vi "ToDatagram.vi"(8 "error in (no error)":errorcluster, 10 "messageID":u16, 11 "PublishMqttMsg in":refnum<class "PublishMqttMsg.lvclass">) -> (0 "error out":errorcluster, 2 "Datagram":u8[](array[numeric]), 3 "PublishMqttMsg out":refnum<class "PublishMqttMsg.lvclass">)   [LabVIEW 2020, in "PublishMqttMsg.lvclass"]
uses:
  PublishMqttMsg.lvclass
  PublishMqttMsg.lvclass/PublishMqttMsg.ctl
  mqttTypedef/mqttMessageType.ctl
  mqtt.lvclass
  BaseMqttMsg.lvclass
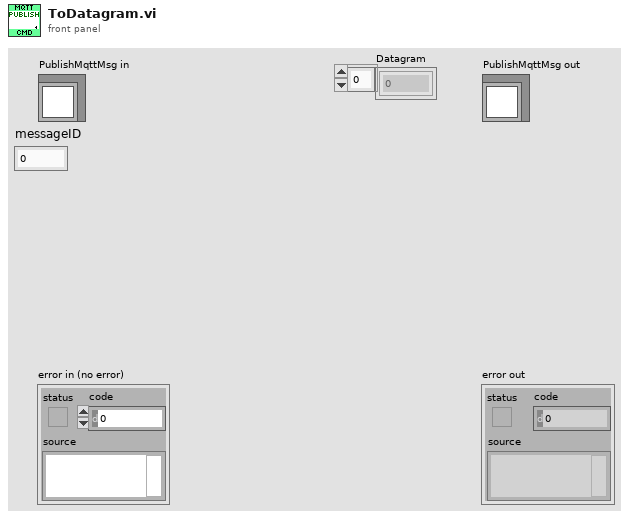
[diagram p1: front panel]
types:
  T1 = typedef "mqtt.lvclass/mqttConnectionMeta.ctl" = cluster{"qos":T2, "duplicate":bool, "retain":bool}
  T2 = typedef "mqtt.lvclass/mqttQOSlevel.ctl" = enum8{"At most once", "At least once", "Exactly once", "Reserved"}
  T3 = typedef "mqtt.lvclass/mqttMessageType.ctl" = enum32{"Reserved", "CONNECT", "CONNACK", "PUBLISH", "PUBACK", "PUBREC", "PUBREL", "PUBCOMP", "SUBSCRIBE", "SUBACK", "UNSUBSCRIBE", "UNSUBACK", "PINGREQ", "PINGRESP", "DISCONNECT", "Reserved2"}
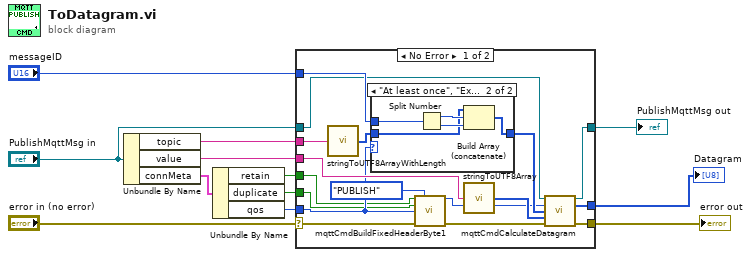
[diagram p0: block diagram]
diagram:
  n1 = Unbundle By Name("PublishMqttMsg in") -> ("topic"=w3:string, "value"=w2:string, "connMeta"=w1:T1)
  n2 = Unbundle By Name(w1) -> ("retain"=w12:bool, "duplicate"=w11:bool, "qos"=w10:T2)
  n3 = case shown="No Error" "error in (no error)" {
    selector: "error in (no error)" -> [w17 w37]
    tunnel: [w13 w37] -> w7
    tunnel: [w20 w36] -> w9
    tunnel: "PublishMqttMsg in" -> [w19 w36]
    tunnel: w3 -> [w27 _]
    tunnel: w2 -> [w29 _]
    tunnel: w10 -> [w21 _]
    tunnel: "messageID" -> [w26 _]
    tunnel: w12 -> [w16 _]
    tunnel: w11 -> [w15 _]
    tunnel: [w14 _] -> w5
    frame No Error {
      n4 = call "stringToUTF8ArrayWithLength.vi"("string"=w27) -> ("UTF8[]"=w28:u8[])  [unwired: 14 in]
      n5 = case shown="\"At least once\", \"Exactly once\"" w21 {
        tunnel: w26 -> [_ w33]
        tunnel: [w30 w32] -> w23
        tunnel: w28 -> [w30 w31]
        frame "At most once", Default {
        }
        frame "At least once", "Exactly once" {
          n6 = Split Number(x=w33) -> (hi(x)=w34:u8, lo(x)=w35:u8)
          n7 = Build Array (concatenate)(w31, w34, w35) -> (w32:u8[])
        }
      }
      n8 = call "mqttCmdBuildFixedHeaderByte1.vi"("retain(F)"=w16, "MessageType"=mqttMessageType."PUBLISH", "duplicate(F)"=w15, "QoS (At most once)"=w21, "error in (no error)"=w17) -> ("byte1"=w22:u8, "error out"=w18:errorcluster)  [unwired: 9 in]
      n9 = call "stringToUTF8Array.vi"("string"=w29) -> ("UTF8[]"=w24:u8[])  [unwired: 14 in]
      n10 = call-dynamic "mqttCmdCalculateDatagram.vi"("mqttCmd in"=w19, "FixedHeaderByte1"=w22, "variableHeader"=w23, "payload"=w24, "error in (no error)"=w18) -> ("mqttCmd out"=w20:refnum<class "PublishMqttMsg.lvclass">, "Datagram"=w14:u8[], "error out"=w13:errorcluster)  [unwired: 8 in]
    }
    frame Error {
    }
  }
  "error out" <- w7
  "PublishMqttMsg out" <- w9
  "Datagram" <- w5
